vi "OAT Compensation filter design for CIC filter (for narrow band filter design).vi"(2 "stop band attenuation":T1(ring)=enum."72 dB", 3 "M":i32=32) -> (0 "CIC stages":i32=9, 1 "filter coefficients":dbl[](graph))   [LabVIEW 2017, in "SoundVib_Resampling.lvlib"]
uses:
  <vilib>/addons/Sound and Vibration/Order Analysis/Resample Order Tracking/SoundVib_Resampling.lvlib
  <vilib>/Analysis/1siggen.llb/Ramp Pattern by Samples.vi
  <vilib>/Analysis/NI_AALBase.lvlib
panel:
  in  "debug?":bool
  out "h":dbl[](array[numeric]) format="%.2f"
  in  "pass band length(0..0.1)":dbl=0.013 format="%.4f"
  in  "WEIGHT":dbl=0.1 format="%.2f"
  out "pass band error":dbl[](graph)
  in  "#of compensation points":i32=30
  in  "linear/log":bool
  out "frequency response":cluster{"Element Data":dbl, dbl, dbl[]}(graph)={"Element Data"=0.0, 1.52587890625e-05, []}
  out "error":i32
  out "ripple":dbl=1.0393984755515295e-07 format="%.2e"
  # "Decimation by two, 1/16 aliasing protection"
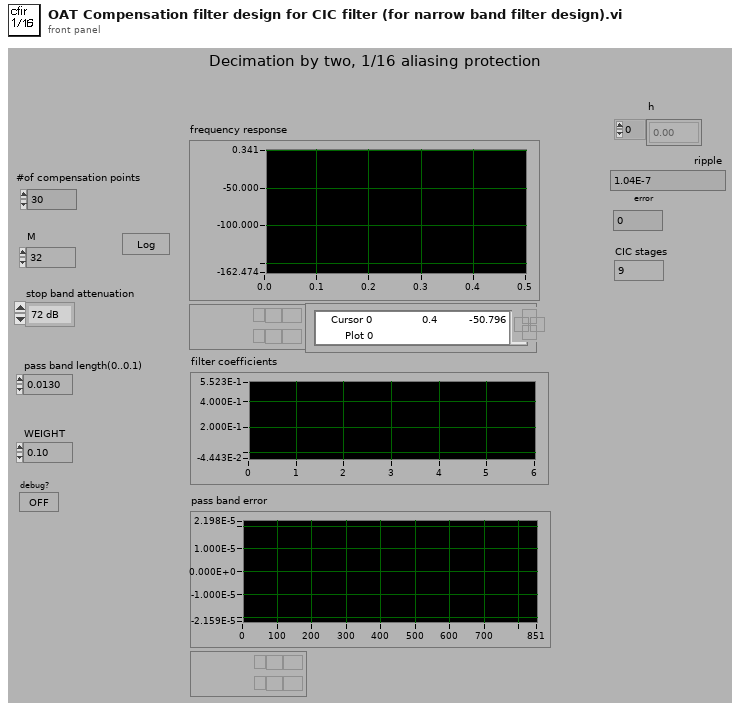
[diagram p1: front panel]
types:
  T1 = enum16{"48 dB", "60 dB", "72 dB", "84 dB", "96 dB", "108 dB", "120 dB"}
  T2 = cluster{"Element Data":dbl, dbl, "Element Data":dbl, "WEIGHT":dbl}
  T3 = cluster{"Element Data":dbl, dbl, "Element Data":dbl, "WEIGHT":dbl}[]
  T4 = cluster{"Element Data":dbl, "df":dbl, "amplitude":dbl[]}
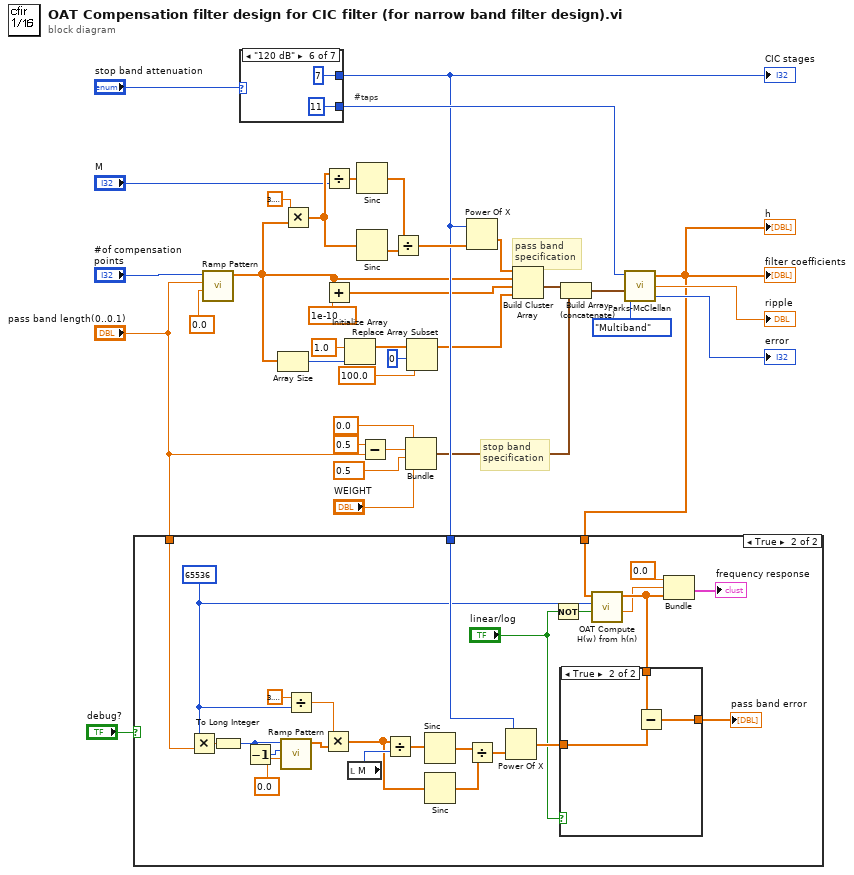
[diagram p0: block diagram]
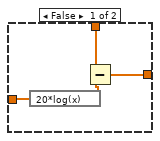
[diagram p3: hidden frame]
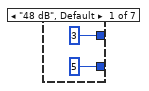
[diagram p4: hidden frame]
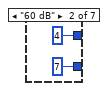
[diagram p5: hidden frame]
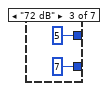
[diagram p6: hidden frame]
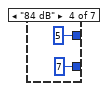
[diagram p7: hidden frame]
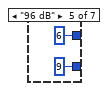
[diagram p8: hidden frame]
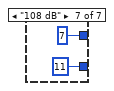
[diagram p9: hidden frame]
diagram:
  # "pass band \nspecification"
  # "stop band \nspecification"
  # "#taps"
  n1 = call-poly <vilib>:"Ramp Pattern.vi"("start"=0.0, "end"="pass band length(0..0.1)", "samples"="#of compensation points") -> ("Ramp Pattern"=w4:dbl[])  [unwired: 7 in, 1 out]
  n2 = case shown="\"120 dB\"" "stop band attenuation" {
    tunnel: [5 7 7 7 9 11 11] -> w26
    tunnel: [3 4 5 5 6 7 7] -> w17
    frame "48 dB", Default {
    }
    frame "60 dB" {
    }
    frame "72 dB" {
    }
    frame "84 dB" {
    }
    frame "96 dB" {
    }
    frame "120 dB" {
    }
    frame "108 dB" {
    }
  }
  "CIC stages" <- w17
  n3 = Array Size(array=w4) -> (size(s)=w13:i32)
  n4 = Multiply(x=3.141592653589793, y=w4) -> (x*y=w24:dbl[])
  n5 = Divide(x=w24, y="M") -> (x/y=w25:dbl[])
  n6 = Add(x=w4, y=1e-10 ("Element Data")) -> (x+y=w5:dbl[])
  n7 = Initialize Array(1.0 ("Element Data"), w13) -> (w12:dbl[])
  n8 = Sinc(1:w25) -> (0:w23:dbl[])
  n9 = Sinc(1:w24) -> (0:w22:dbl[])
  n10 = Subtract(x=0.5, y="pass band length(0..0.1)") -> (x-y=w8:dbl)
  n11 = Divide(x=w23, y=w22) -> (x/y=w18:dbl[])
  n12 = Bundle("Element Data"=0.0, w8, "Element Data"=0.5, "WEIGHT"="WEIGHT") -> (w2:T2)  [unwired: 1 in]
  n13 = Replace Array Subset(array=w12, new element=100.0 ("Element Data"), index=0 ("Index")) -> (w10:dbl[])
  n14 = Power Of X(1:w18, 2:w17) -> (0:w14:dbl[])
  n15 = Build Cluster Array(w14, w4, w5, w10) -> (w3:cluster{dbl, dbl, dbl, "Element Data":dbl}[])
  n16 = Build Array (concatenate)(w3, w2) -> (w1:T3)
  n17 = call <vilib>:"Parks-McClellan.vi"("filter type"=enum32{"Multiband", "Differentiator", "Hilbert"}."Multiband", "Band Parameters"=w1, "# of taps"=w26) -> ("error"=→"error":i32, "ripple"=→"ripple":dbl, "h"=w28:dbl[])  [unwired: 1 in]
  "filter coefficients" <- w28
  "h" <- w28
  n18 = case shown="True" "debug?" {
    tunnel: w28 -> [_ w70]
    tunnel: "pass band length(0..0.1)" -> [_ w65]
    tunnel: w17 -> [_ w71]
    frame False {
    }
    frame True {
      w61 = 65536 ("Element Data")
      n19 = Multiply(x=w61, y=w65) -> (x*y=w64:dbl)
      n20 = To Long Integer(number=w64) -> (32bit integer=w63:i32)
      n21 = Decrement(x=w63) -> (x-1=w62:i32)
      n22 = call-poly <vilib>:"Ramp Pattern.vi"("start"=0.0, "end"=w62, "samples"=w63) -> ("Ramp Pattern"=w55:dbl[])  [unwired: 7 in, 1 out]
      n23 = Divide(x=3.141592653589793, y=w61) -> (x/y=w54:dbl)
      n24 = Multiply(x=w54, y=w55) -> (x*y=w52:dbl[])
      n25 = local read "M"() -> (w53:i32)
      n26 = Divide(x=w52, y=w53) -> (x/y=w57:dbl[])
      n27 = Sinc(1:w57) -> (0:w58:dbl[])
      n28 = Sinc(1:w52) -> (0:w59:dbl[])
      n29 = Divide(x=w58, y=w59) -> (x/y=w51:dbl[])
      n30 = Power Of X(1:w51, 2:w71) -> (0:w72:dbl[])
      n31 = Not(x="linear/log") -> (.not. x?=w66:bool)
      n32 = call <vilib>:"OAT Compute H(w) from h(n).vi"("dB on?"=w66, "number of frequicies"=w61, "h[n]"=w70) -> ("df"=w68:dbl, "amplitude"=w69:dbl[])  [unwired: 6 in, 1 out]
      n33 = case shown="True" "linear/log" {
        tunnel: [w76 w80] -> w73
        tunnel: w69 -> [w78 w82]
        tunnel: w72 -> [w79 w81]
        frame False {
          n34 = expression code="20*log(x)"(w79) -> (w77:dbl[])
          n35 = Subtract(x=w78, y=w77) -> (x-y=w76:dbl[])
        }
        frame True {
          n36 = Subtract(x=w82, y=w81) -> (x-y=w80:dbl[])
        }
      }
      "pass band error" <- w73
      n37 = Bundle("Element Data"=0.0, "df"=w68, "amplitude"=w69) -> (→"frequency response":T4)  [unwired: 1 in]
    }
  }
